vi "onTestSlippage.vi"(7 "Project in":refnum<class "RequirementMap.lvclass">, 11 "Leaf.TestCase":refnum<class "Leaf.TestCase.lvclass">) -> (0 "error out":errorcluster, 3 "Leaf.TestCase":refnum<class "Leaf.TestCase.lvclass">)   [LabVIEW 2021, in "Bananas.lvlib" / "RequirementMap.lvclass"]
uses:
  RequirementMap.lvclass
  Leaf.TestCase/Leaf.TestCase.lvclass
  C:/Repositories/LVOS/Bananas/lv-src/Bananas/Leaf/Leaf.lvclass
  RequirementMap.lvclass/RequirementMap.ctl
  Leaf/Leaf.lvclass
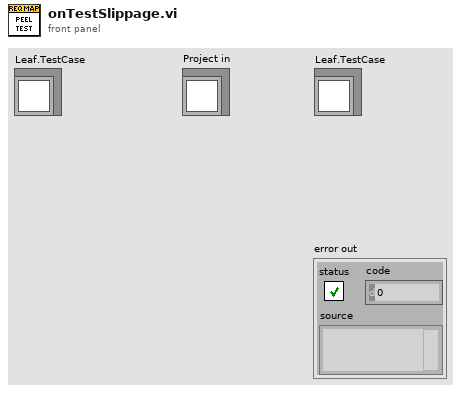
[diagram p1: front panel]
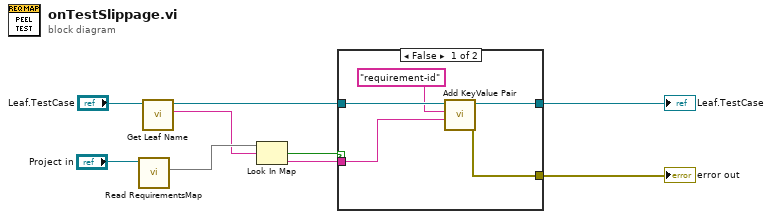
[diagram p0: block diagram]
diagram:
  n1 = call "Read RequirementsMap.vi"("RequirementsFile in"="Project in") -> ("Requirements"=w9:map{string, string})  [unwired: 9 in, 1 out]
  n2 = call "Get Leaf Name.vi"("Leaf in"="Leaf.TestCase") -> ("Name"=w2:string, "Leaf out"=w3:refnum<class "Leaf.TestCase.lvclass">)  [unwired: 8 in, 1 out]
  n3 = Look In Map(map=w9, key=w2) -> (key not found?=w8:bool, value=w7:string)  [unwired: 1 in]
  n4 = case shown="False" w8 {
    tunnel: [w11 w15] -> w5
    tunnel: w3 -> [w13 w15]
    tunnel: w7 -> [w14 _]
    tunnel: [w10 _] -> w4
    frame False {
      n5 = call "Add KeyValue Pair.vi"("value"=w14, "key"="requirement-id", "Leaf in"=w13) -> ("error out"=w10:errorcluster, "Leaf out"=w11:refnum<class "Leaf.TestCase.lvclass">)  [unwired: 7 in]
    }
    frame True {
    }
  }
  "error out" <- w4
  "Leaf.TestCase" <- w5
